vi "PLC.vi"(7 "Notifiers":T4, 8 "error in":errorcluster, 11 "Message Queues":T3) -> (0 "error out":errorcluster)   [LabVIEW 2014]
uses:
  Message Queue/Message Queue.lvlib
  Message Queue/Enqueue Message (Single).vi
  PL Model/PL Model.lvlib
  <vilib>/Utility/error.llb/Error Cluster From Error Code.vi
  Logger/Logger.lvlib
  <vilib>/ErrorRing/Error Ring.xnode
  DAQ/DAQ.lvlib
  TCP/TCP.lvlib
  Exit Notifiers/PLC Notifiers.ctl
  Exit Notifiers/PLC Notifiers.lvlib
  Message Queue/Message Cluster.ctl
  Message Queue/All Message Queues.ctl
  DAQ/TypeDefs/DAQ data.ctl
  controls/PLC Data.ctl
panel:
  in  "PLC Data":T1
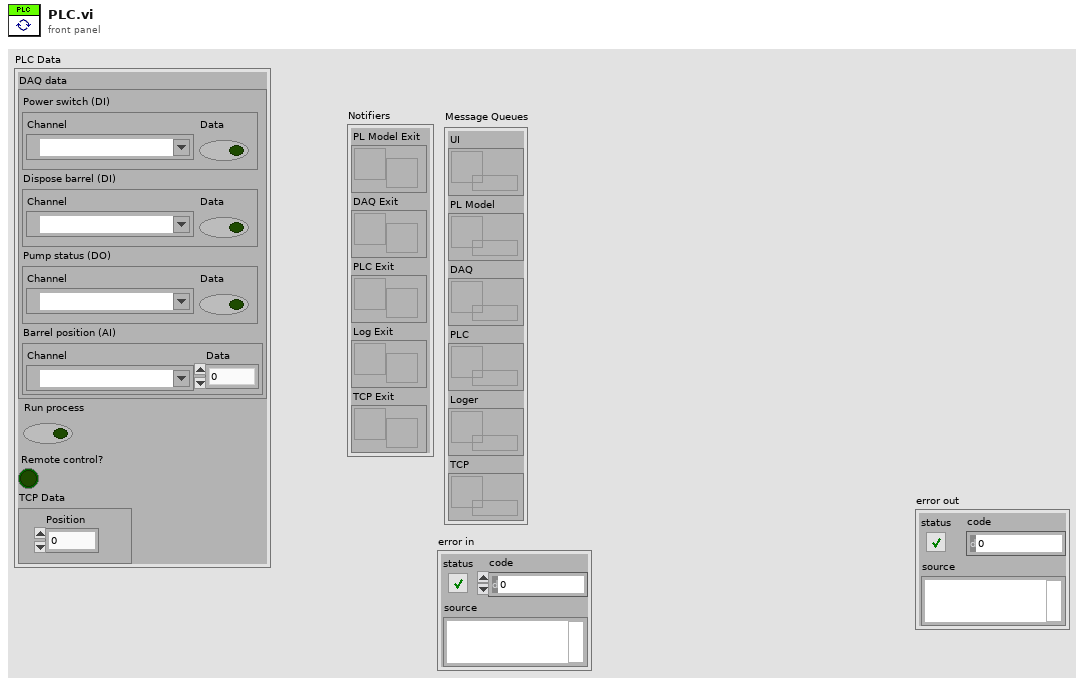
[diagram p1: front panel]
types:
  T1 = typedef "PLC Data.ctl" = cluster{"DAQ data":T2, "Run process":bool, "Remote control?":bool, "TCP Data":cluster{"Position":dbl}}
  T2 = typedef "DAQ.lvlib/DAQ data.ctl" = cluster{"Power switch (DI)":cluster{"Channel":tag, "Data":bool}, "Dispose barrel (DI)":cluster{"Channel":tag, "Data":bool}, "Pump status (DO)":cluster{"Channel":tag, "Data":bool}, "Barrel position (AI)":cluster{"Channel":tag, "Data":dbl}}
  T3 = typedef "Message Queue.lvlib/All Message Queues.ctl" = cluster{"UI":refnum<queue>, "PL Model":refnum<queue>, "DAQ":refnum<queue>, "PLC":refnum<queue>, "Loger":refnum<queue>, "TCP":refnum<queue>}
  T4 = typedef "PLC Notifiers.lvlib/PLC Notifiers.ctl" = cluster{"PL Model Exit":refnum<notifier>, "DAQ Exit":refnum<notifier>, "PLC Exit":refnum<notifier>, "Log Exit":refnum<notifier>, "TCP Exit":refnum<notifier>}
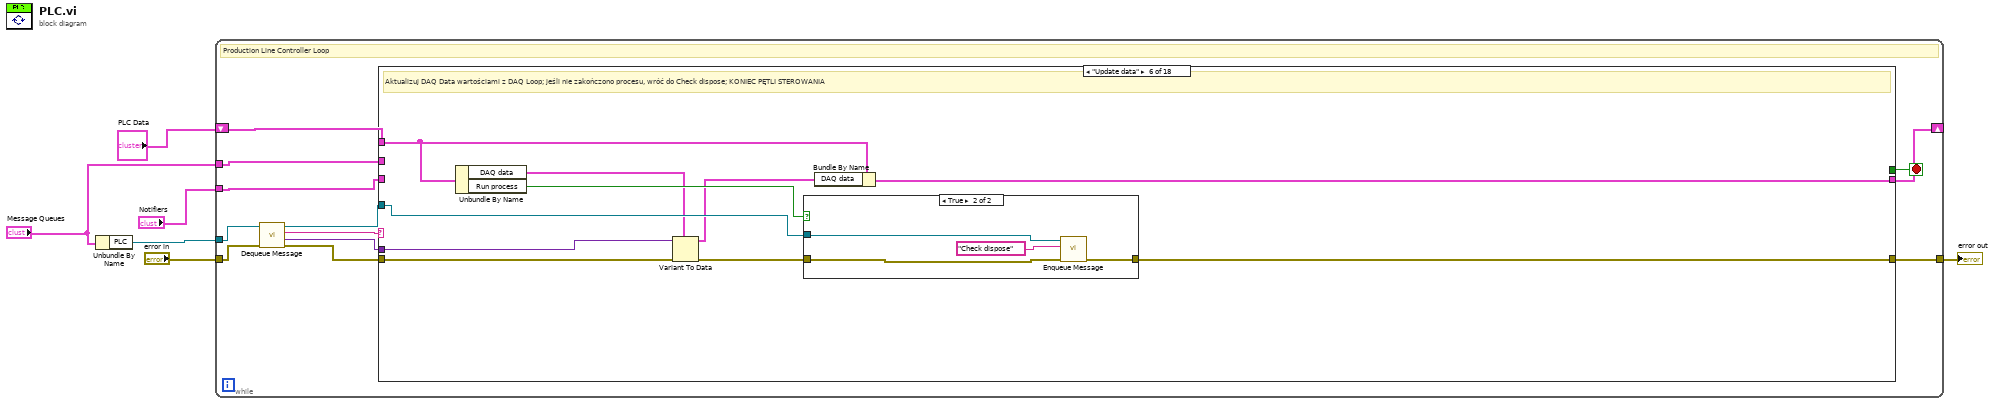
[diagram p0: block diagram]
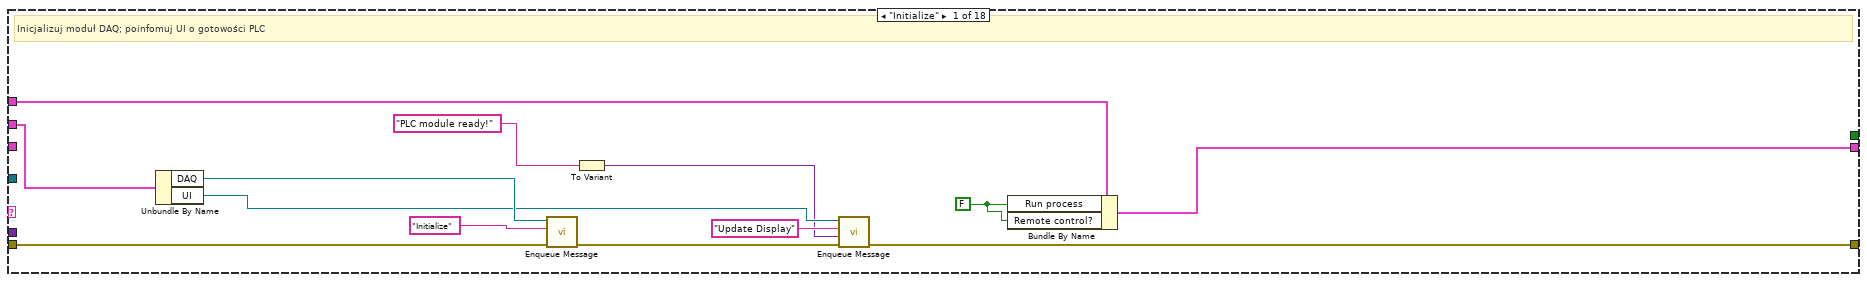
[diagram p2: hidden frame]
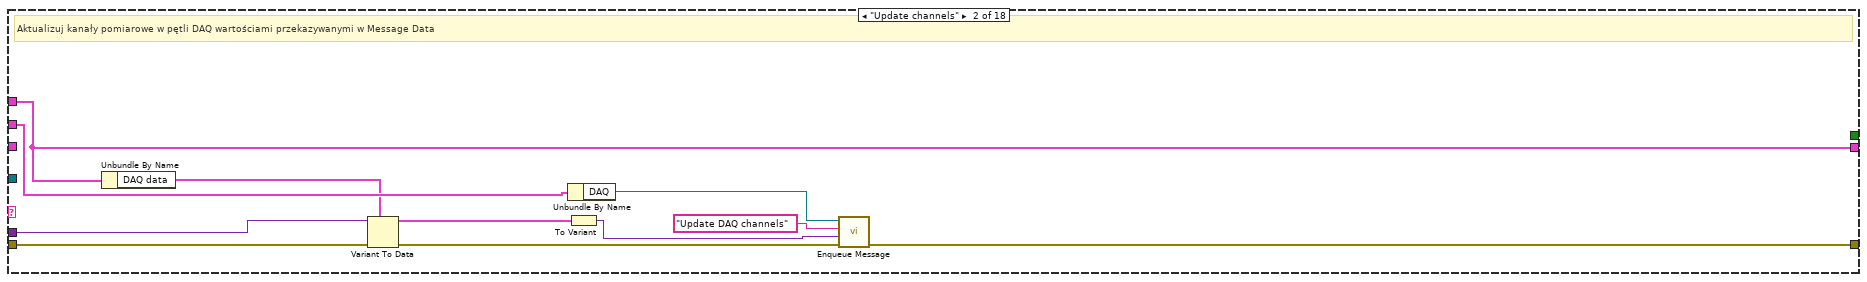
[diagram p3: hidden frame]
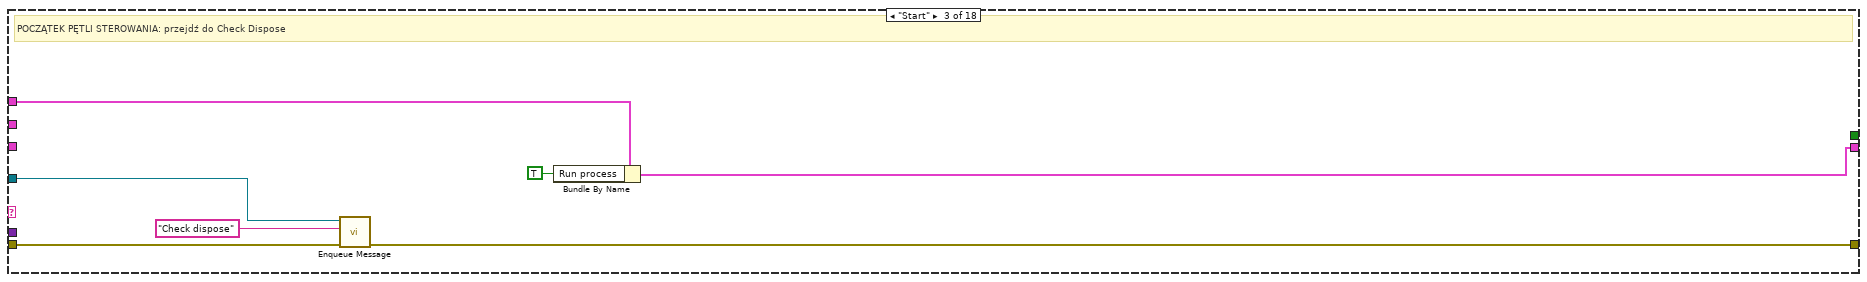
[diagram p4: hidden frame]
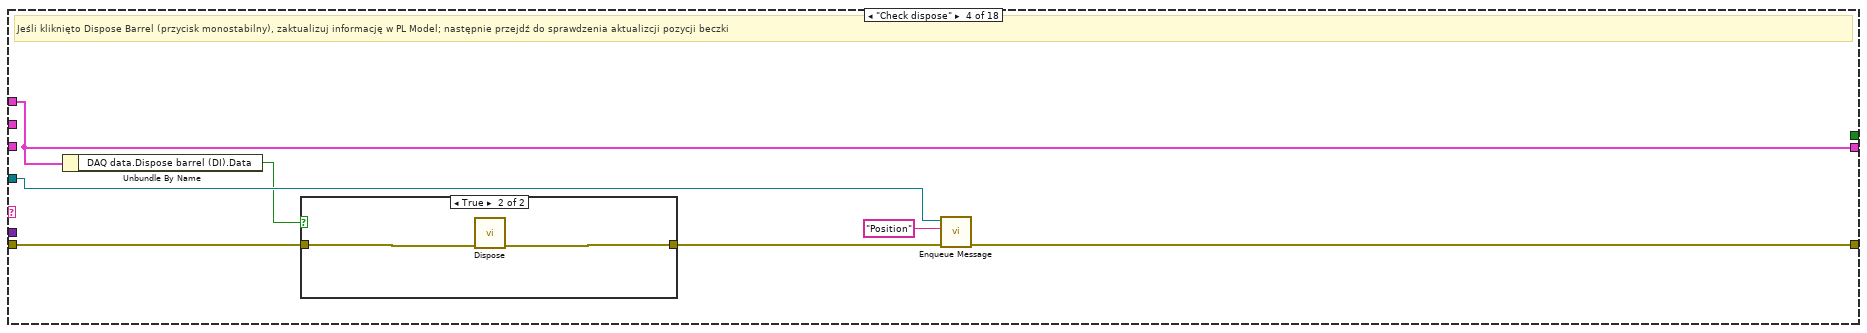
[diagram p5: hidden frame]
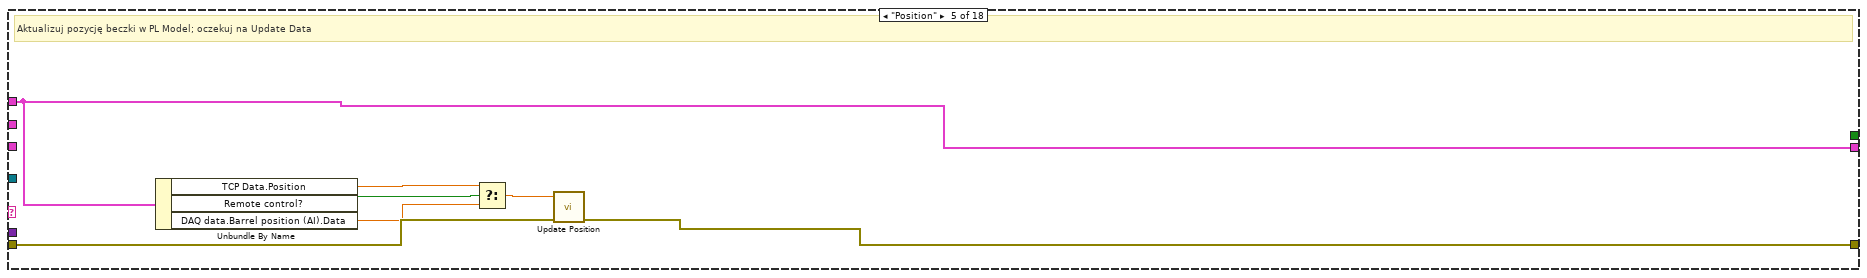
[diagram p7: hidden frame]
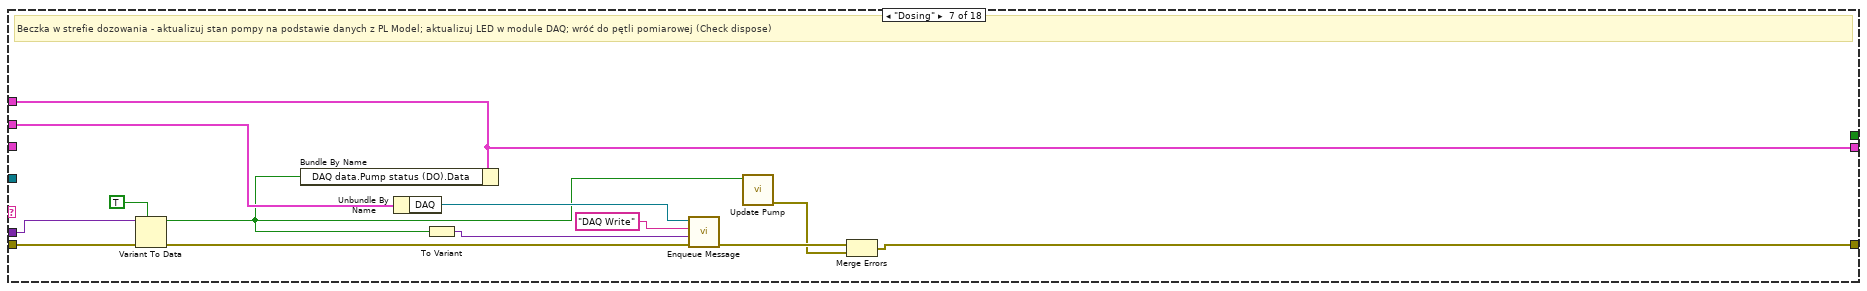
[diagram p9: hidden frame]
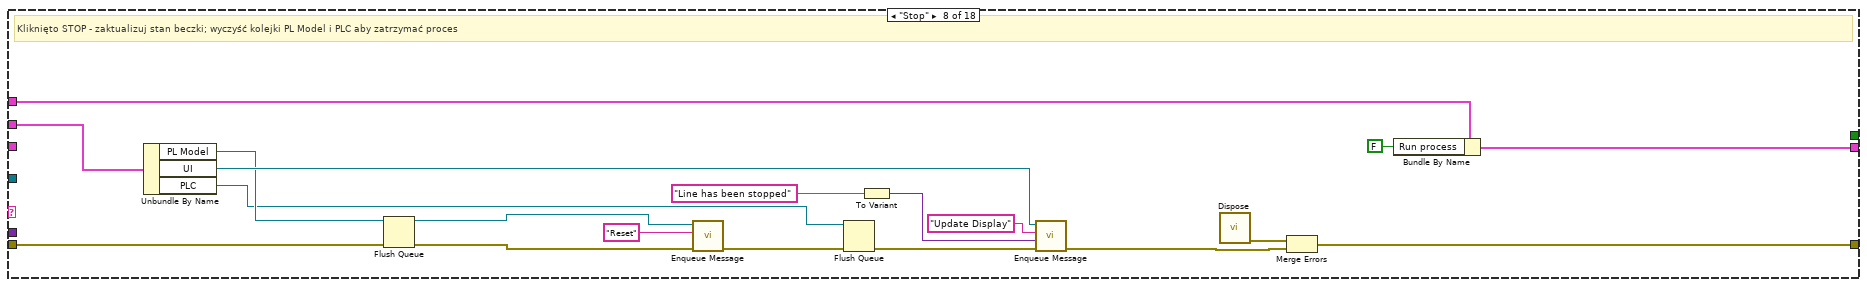
[diagram p10: hidden frame]
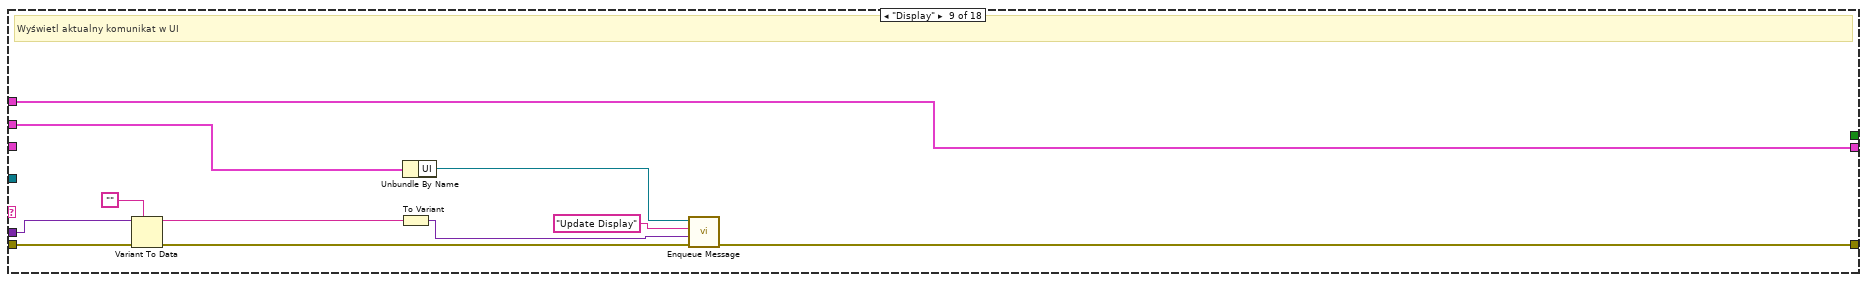
[diagram p11: hidden frame]
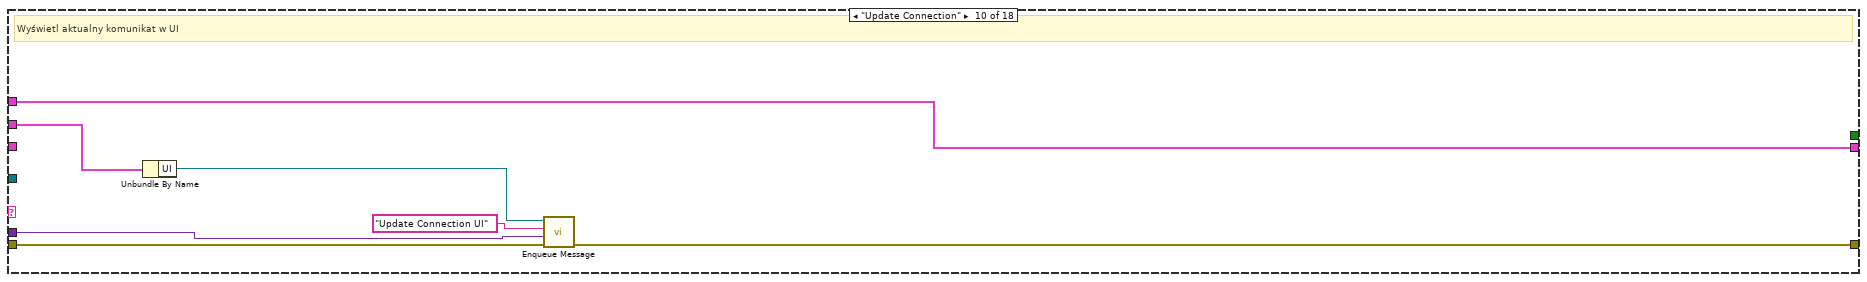
[diagram p12: hidden frame]
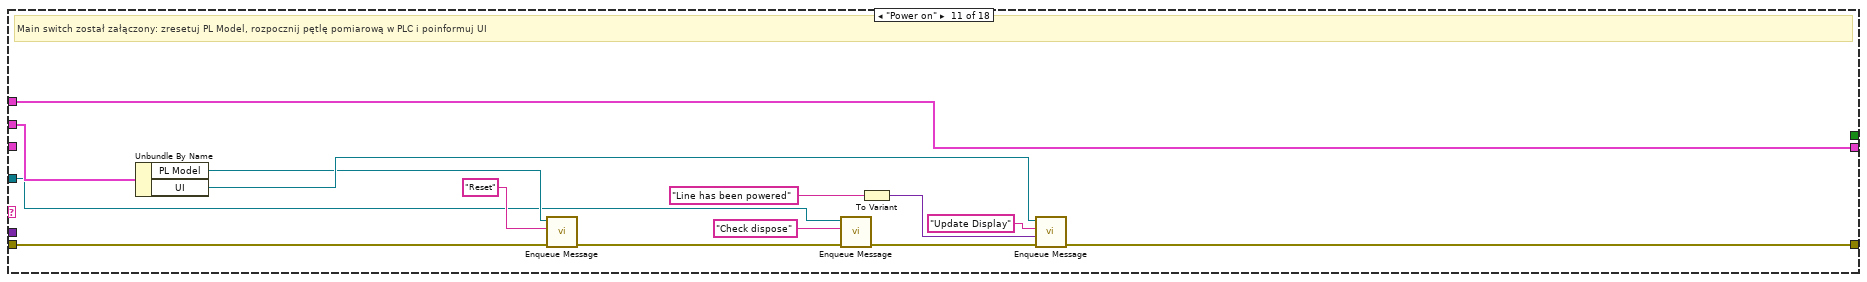
[diagram p13: hidden frame]
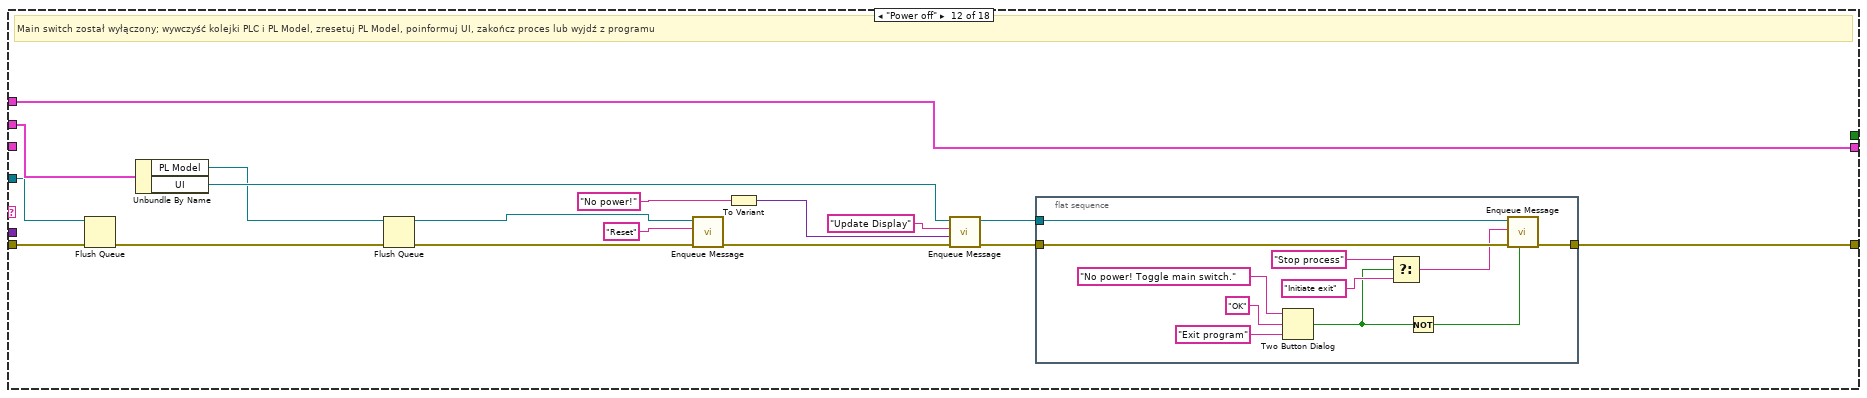
[diagram p14: hidden frame]
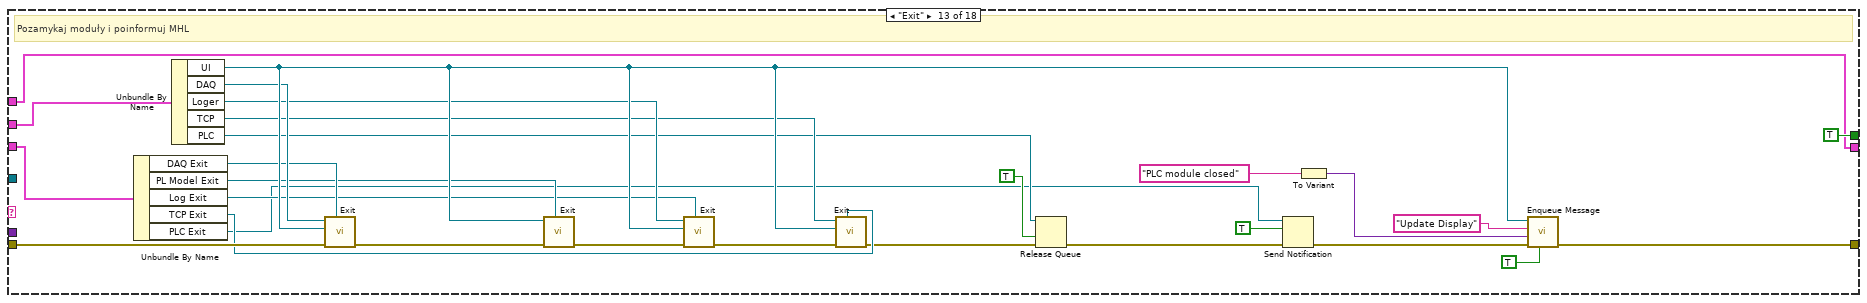
[diagram p15: hidden frame]
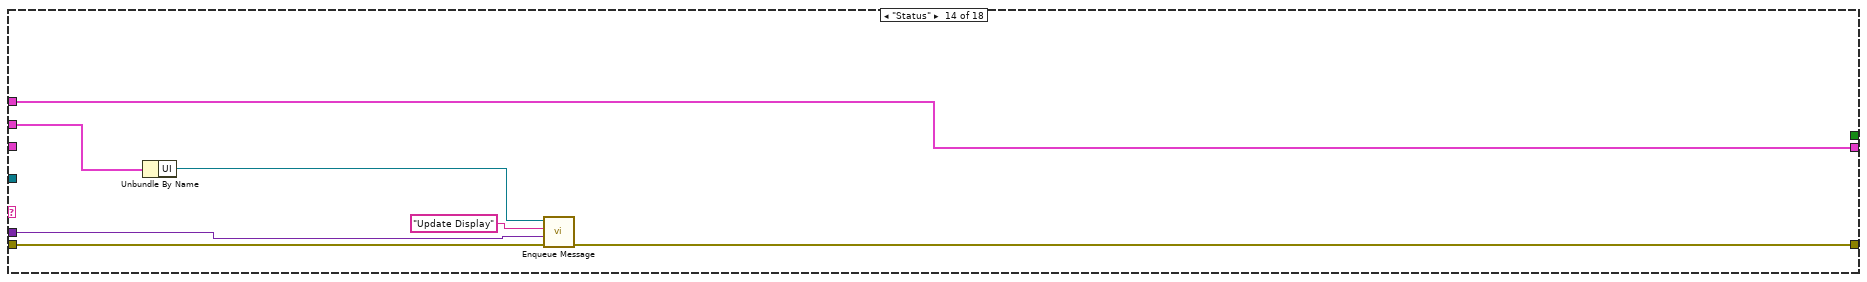
[diagram p16: hidden frame]
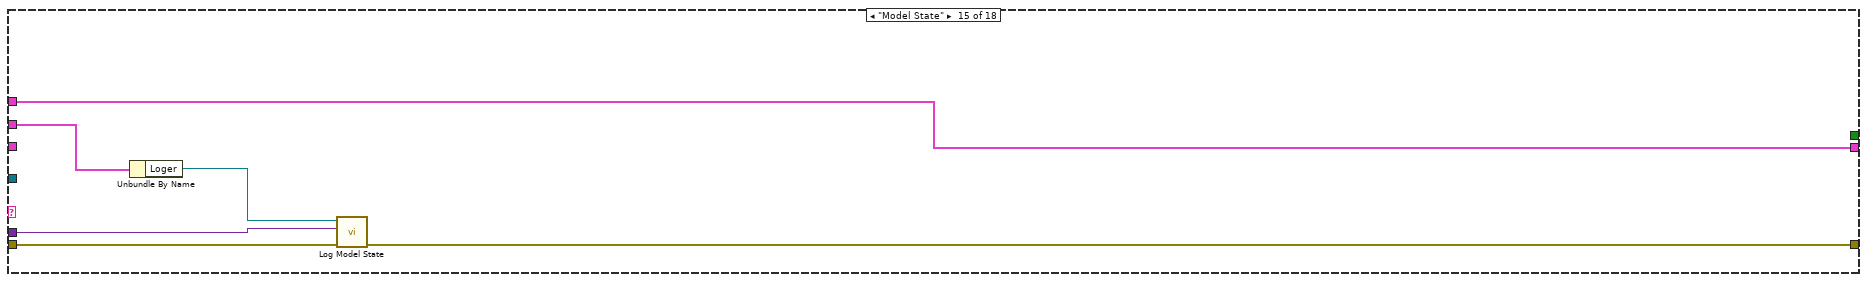
[diagram p17: hidden frame]
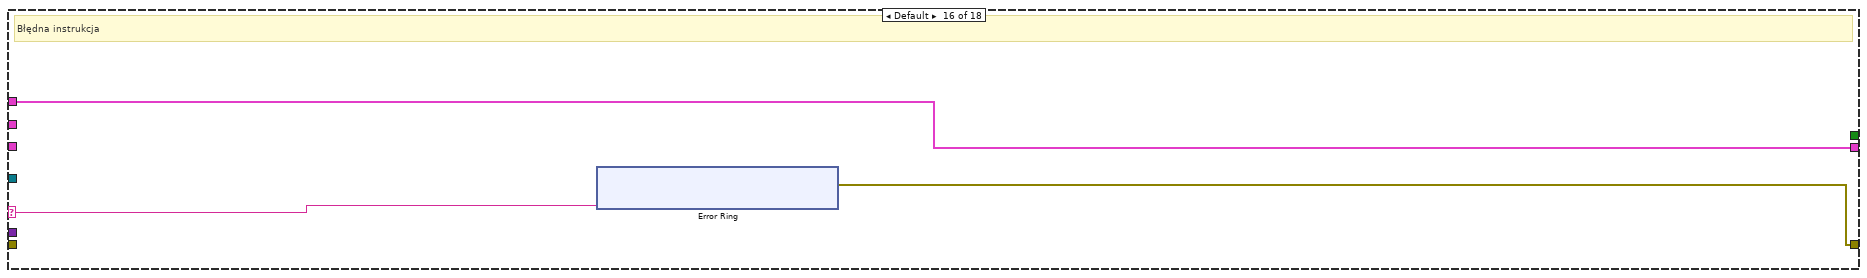
[diagram p18: hidden frame]
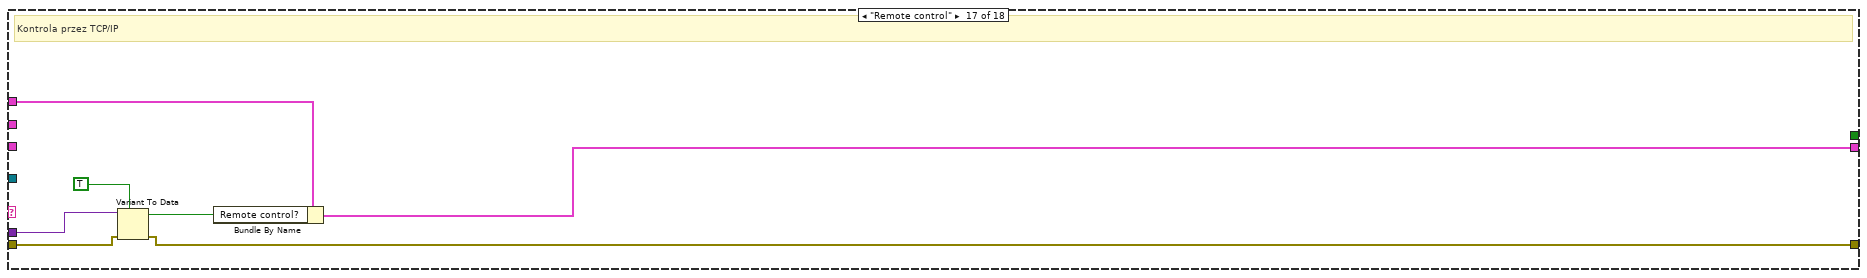
[diagram p19: hidden frame]
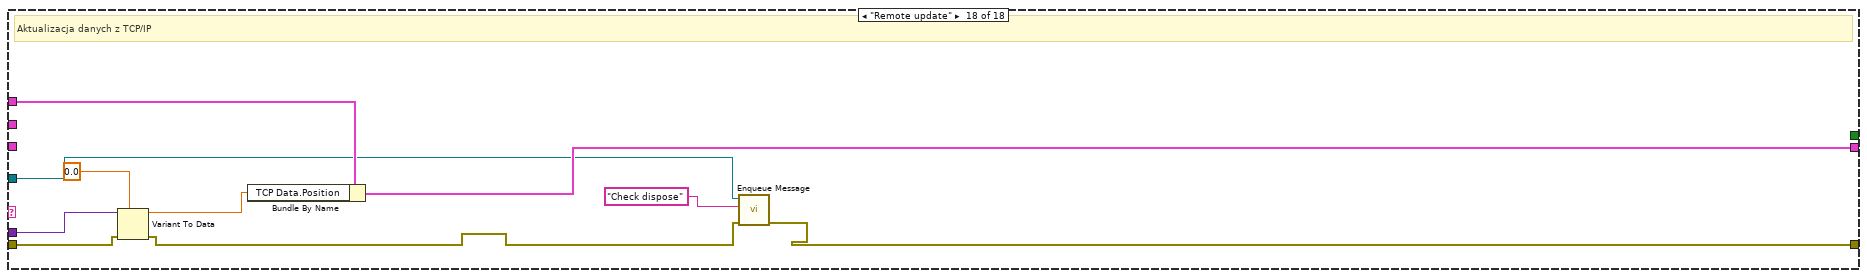
[diagram p20: hidden frame]
diagram:
  n1 = Unbundle By Name("Message Queues") -> ("PLC"=w3:refnum<queue>)
  n2 = while {
    tunnel: "Notifiers" -> [w17]
    tunnel: w3 -> [w16]
    tunnel: "error in" -> [w15]
    tunnel: [w12] -> w5
    tunnel: "Message Queues" -> [w11]
    shift-right: [w9] -> _
    shift-left: "PLC Data" -> [w8]
    stop <- w13 stop-if-true
    # "Production Line Controller Loop"
    n3 = call "Dequeue Message.vi"("error in (no error)"=w15, "Message Queue"=w16) -> ("error out"=w14:errorcluster, "Message Data"=w10:variant, "Message"=w18:string, "dup Message Queue"=w7:refnum<queue>)  [unwired: 6 in]
    n4 = case shown="\"Update data\"" w18 {
      selector: w18 -> [_ _ _ _ _ _ _ _ _ _ _ _ _ _ _ w216 _ _]
      tunnel: w17 -> [_ _ _ _ _ _ _ _ _ _ _ _ w196 _ _ _ _ _]
      tunnel: w14 -> [w30 w41 w43 w53 w66 w75 w90 w109 w120 w125 w139 w153 w199 w206 w211 _ w231 w241]
      tunnel: w7 -> [_ _ w48 w56 _ w74 _ _ _ _ w137 w154 _ _ _ _ _ w232]
      tunnel: [_ _ _ _ _ _ _ _ _ _ _ _ TRUE _ _ _ _ _] -> w13
      tunnel: [w24 w36 w47 w54 w60 w72 w82 w96 w122 w129 w133 w157 w174 w202 w209 w215 w225 w233] -> w12
      tunnel: w11 -> [w31 w38 _ _ _ _ w94 w113 w124 w131 w143 w162 w197 w207 w213 _ _ _]
      tunnel: w10 -> [_ w42 _ _ _ w76 w89 _ w121 w126 _ _ _ w204 w210 _ w230 w240]
      tunnel: w8 -> [w21 w33 w46 w50 w65 w71 w91 w104 w114 w127 w132 w146 w200 w208 w214 w217 w227 w239]
      tunnel: [w20 w33 w45 w50 w65 w70 w91 w102 w114 w127 w132 w146 w200 w208 w214 w217 w226 w238] -> w9
      frame "Initialize" {
        w19 = FALSE ("Run process")
        # "Inicjalizuj moduł DAQ; poinfomuj UI o gotowości PLC"
        n5 = Unbundle By Name(w31) -> ("DAQ"=w29:refnum<queue>, "UI"=w23:refnum<queue>)
        n6 = call-poly "Enqueue Message.vi"("error in (no error)"=w30, "Message"="Initialize", "Message Queue"=w29) -> ("error out"=w25:errorcluster)  [unwired: 7 in, 1 out]
        n7 = To Variant(anything="PLC module ready!" ("Message")) -> (Variant=w22:variant)
        n8 = call-poly "Enqueue Message.vi"("error in (no error)"=w25, "Message Data"=w22, "Message"="Update Display", "Message Queue"=w23) -> ("error out"=w24:errorcluster)  [unwired: 6 in, 1 out]
        n9 = Bundle By Name(cluster=w21, "Run process"=w19, "Remote control?"=w19) -> (w20:T1)
      }
      frame "Update channels" {
        # "Aktualizuj kanały pomiarowe w pętli DAQ wartościami przekazywanymi w Message Data"
        n10 = Unbundle By Name(w33) -> ("DAQ data"=w32:T2)
        n11 = Variant To Data(error in=w41, type=w32, Variant=w42) -> (data=w34:T2, error out=w40:errorcluster)
        n12 = Unbundle By Name(w38) -> ("DAQ"=w37:refnum<queue>)
        n13 = To Variant(anything=w34) -> (Variant=w35:variant)
        n14 = call-poly "Enqueue Message.vi"("error in (no error)"=w40, "Message Data"=w35, "Message"="Update DAQ channels", "Message Queue"=w37) -> ("error out"=w36:errorcluster)  [unwired: 6 in, 1 out]
      }
      frame "Start" {
        # "POCZĄTEK PĘTLI STEROWANIA: przejdź do Check Dispose"
        n15 = call-poly "Enqueue Message.vi"("error in (no error)"=w43, "Message"="Check dispose", "Message Queue"=w48) -> ("error out"=w47:errorcluster)  [unwired: 7 in, 1 out]
        n16 = Bundle By Name(cluster=w46, "Run process"=TRUE) -> (w45:T1)
      }
      frame "Check dispose" {
        # "Jeśli kliknięto Dispose Barrel (przycisk monostabilny), zaktualizuj informację w PL Model; następnie przejdź do sprawdzenia aktualizcji pozycji beczki"
        n17 = Unbundle By Name(w50) -> ("DAQ data.Dispose barrel (DI).Data"=w51:bool)
        n18 = case shown="True" w51 {
          tunnel: w53 -> [w57 w59]
          tunnel: [w57 w58] -> w52
          frame False {
          }
          frame True {
            n19 = call "Dispose.vi"("error in (no error)"=w59) -> ("error out"=w58:errorcluster)  [unwired: 10 in]
          }
        }
        n20 = call-poly "Enqueue Message.vi"("error in (no error)"=w52, "Message"="Position", "Message Queue"=w56) -> ("error out"=w54:errorcluster)  [unwired: 7 in, 1 out]
      }
      frame "Position" {
        # "Aktualizuj pozycję beczki w PL Model; oczekuj na Update Data"
        n21 = Unbundle By Name(w65) -> ("TCP Data.Position"=w64:dbl, "Remote control?"=w61:bool, "DAQ data.Barrel position (AI).Data"=w62:dbl)
        n22 = Select(t=w64, s=w61, f=w62) -> (s? t:f=w63:dbl)
        n23 = call "Update Position.vi"("error in (no error)"=w66, "Position"=w63) -> ("error out"=w60:errorcluster)  [unwired: 9 in]
      }
      frame "Update data" {
        # "Aktualizuj DAQ Data wartościami z DAQ Loop; jeśli nie zakończono procesu, wróć do Check dispose; KONIEC PĘTLI STEROWANIA"
        n24 = Unbundle By Name(w71) -> ("DAQ data"=w67:T2, "Run process"=w69:bool)
        n25 = Variant To Data(error in=w75, type=w67, Variant=w76) -> (data=w68:T2, error out=w73:errorcluster)
        n26 = case shown="True" w69 {
          tunnel: w74 -> [_ w80]
          tunnel: w73 -> [w77 w79]
          tunnel: [w77 w78] -> w72
          frame False {
          }
          frame True {
            n27 = call-poly "Enqueue Message.vi"("error in (no error)"=w79, "Message"="Check dispose", "Message Queue"=w80) -> ("error out"=w78:errorcluster)  [unwired: 7 in, 1 out]
          }
        }
        n28 = Bundle By Name(cluster=w71, "DAQ data"=w68) -> (w70:T1)
      }
      frame "Dosing" {
        # "Beczka w strefie dozowania - aktualizuj stan pompy na podstawie danych z PL Model; aktualizuj LED w module DAQ; wróć do pętli pomiarowej (Check dispose)"
        n29 = Variant To Data(error in=w90, type=TRUE, Variant=w89) -> (data=w86:bool, error out=w83:errorcluster)
        n30 = Bundle By Name(cluster=w91, "DAQ data.Pump status (DO).Data"=w86) -> ()  [unwired: 1 out]
        n31 = Unbundle By Name(w94) -> ("DAQ"=w93:refnum<queue>)
        n32 = To Variant(anything=w86) -> (Variant=w87:variant)
        n33 = call-poly "Enqueue Message.vi"("error in (no error)"=w83, "Message Data"=w87, "Message"="DAQ Write", "Message Queue"=w93) -> ("error out"=w85:errorcluster)  [unwired: 6 in, 1 out]
        n34 = call "Update Pump.vi"("Pump State"=w86) -> ("error out"=w84:errorcluster)  [unwired: 10 in]
        n35 = Merge Errors(w85, w84) -> (w82:errorcluster)
      }
      frame "Stop" {
        # "Kliknięto STOP - zaktualizuj stan beczki; wyczyść kolejki PL Model i PLC aby zatrzymać proces"
        n36 = Unbundle By Name(w113) -> ("PL Model"=w110:refnum<queue>, "UI"=w111:refnum<queue>, "PLC"=w108:refnum<queue>)
        n37 = Flush Queue(queue=w110, error in (no error)=w109) -> (queue out=w101:refnum<queue>, error out=w95:errorcluster)  [unwired: 1 out]
        n38 = call-poly "Enqueue Message.vi"("error in (no error)"=w95, "Message"="Reset", "Message Queue"=w101) -> ("error out"=w99:errorcluster)  [unwired: 7 in, 1 out]
        n39 = Flush Queue(queue=w108, error in (no error)=w99) -> (error out=w107:errorcluster)  [unwired: 2 out]
        n40 = To Variant(anything="Line has been stopped" ("Message")) -> (Variant=w105:variant)
        n41 = call-poly "Enqueue Message.vi"("error in (no error)"=w107, "Message Data"=w105, "Message"="Update Display", "Message Queue"=w111) -> ("error out"=w97:errorcluster)  [unwired: 6 in, 1 out]
        n42 = call "Dispose.vi"() -> ("error out"=w98:errorcluster)  [unwired: 11 in]
        n43 = Merge Errors(w98, w97) -> (w96:errorcluster)
        n44 = Bundle By Name(cluster=w104, "Run process"=FALSE) -> (w102:T1)
      }
      frame "Display" {
        # "Wyświetl aktualny komunikat w UI"
        n45 = Variant To Data(error in=w120, type="", Variant=w121) -> (data=w116:string, error out=w119:errorcluster)
        n46 = To Variant(anything=w116) -> (Variant=w115:variant)
        n47 = Unbundle By Name(w124) -> ("UI"=w123:refnum<queue>)
        n48 = call-poly "Enqueue Message.vi"("error in (no error)"=w119, "Message Data"=w115, "Message"="Update Display", "Message Queue"=w123) -> ("error out"=w122:errorcluster)  [unwired: 6 in, 1 out]
      }
      frame "Update Connection" {
        # "Wyświetl aktualny komunikat w UI"
        n49 = Unbundle By Name(w131) -> ("UI"=w130:refnum<queue>)
        n50 = call-poly "Enqueue Message.vi"("error in (no error)"=w125, "Message Data"=w126, "Message"="Update Connection UI", "Message Queue"=w130) -> ("error out"=w129:errorcluster)  [unwired: 6 in, 1 out]
      }
      frame "Power on" {
        # "Main switch został załączony: zresetuj PL Model, rozpocznij pętlę pomiarową w PLC i poinformuj UI"
        n51 = Unbundle By Name(w143) -> ("PL Model"=w140:refnum<queue>, "UI"=w142:refnum<queue>)
        n52 = call-poly "Enqueue Message.vi"("error in (no error)"=w139, "Message"="Reset", "Message Queue"=w140) -> ("error out"=w136:errorcluster)  [unwired: 7 in, 1 out]
        n53 = call-poly "Enqueue Message.vi"("error in (no error)"=w136, "Message"="Check dispose", "Message Queue"=w137) -> ("error out"=w134:errorcluster)  [unwired: 7 in, 1 out]
        n54 = To Variant(anything="Line has been powered" ("Message")) -> (Variant=w141:variant)
        n55 = call-poly "Enqueue Message.vi"("error in (no error)"=w134, "Message Data"=w141, "Message"="Update Display", "Message Queue"=w142) -> ("error out"=w133:errorcluster)  [unwired: 6 in, 1 out]
      }
      frame "Power off" {
        # "Main switch został wyłączony; wywczyść kolejki PLC i PL Model, zresetuj PL Model, poinformuj UI, zakończ proces lub wyjdź z programu"
        n56 = Flush Queue(queue=w154, error in (no error)=w153) -> (error out=w152:errorcluster)  [unwired: 2 out]
        n57 = Unbundle By Name(w162) -> ("PL Model"=w151:refnum<queue>, "UI"=w161:refnum<queue>)
        n58 = Flush Queue(queue=w151, error in (no error)=w152) -> (queue out=w150:refnum<queue>, error out=w149:errorcluster)  [unwired: 1 out]
        n59 = call-poly "Enqueue Message.vi"("error in (no error)"=w149, "Message"="Reset", "Message Queue"=w150) -> ("error out"=w147:errorcluster)  [unwired: 7 in, 1 out]
        n60 = To Variant(anything="No power!" ("Message")) -> (Variant=w155:variant)
        n61 = call-poly "Enqueue Message.vi"("error in (no error)"=w147, "Message Data"=w155, "Message"="Update Display", "Message Queue"=w161) -> ("error out"=w158:errorcluster, "dup Message Queue"=w156:refnum<queue>)  [unwired: 6 in]
        n62 = flat-sequence {
          tunnel: w158 -> [w170]
          tunnel: [w169] -> w157
          tunnel: w156 -> [w168]
          frame #0 {
            n63 = Two Button Dialog(message="No power! Toggle main switch.", 1:"Exit program" ("F button name (\"Cancel\")"), 2:"OK" ("button name (\"OK\")")) -> (T button?=w164:bool)
            n64 = Select(t="Stop process" ("Message"), s=w164, f="Initiate exit" ("Message")) -> (s? t:f=w165:string)
            n65 = Not(x=w164) -> (.not. x?=w163:bool)
            n66 = call-poly "Enqueue Message.vi"("Priority Message? (F)"=w163, "error in (no error)"=w170, "Message"=w165, "Message Queue"=w168) -> ("error out"=w169:errorcluster)  [unwired: 6 in, 1 out]
          }
        }
      }
      frame "Exit" {
        # "Pozamykaj moduły i poinformuj MHL"
        n67 = Unbundle By Name(w196) -> ("DAQ Exit"=w181:refnum<notifier>, "PL Model Exit"=w180:refnum<notifier>, "Log Exit"=w179:refnum<notifier>, "TCP Exit"=w178:refnum<notifier>, "PLC Exit"=w177:refnum<notifier>)
        n68 = Unbundle By Name(w197) -> ("UI"=w186:refnum<queue>, "DAQ"=w185:refnum<queue>, "Loger"=w184:refnum<queue>, "TCP"=w183:refnum<queue>, "PLC"=w182:refnum<queue>)
        n69 = call "Exit.vi"("Exit Notifier"=w181, "error in"=w199, "UI Queue"=w186, "Message Queue"=w185) -> ("error out"=w195:errorcluster)  [unwired: 7 in]
        n70 = call "Exit.vi"("Exit Notifier"=w180, "error in (no error)"=w195, "UI Queue"=w186) -> ("error out"=w198:errorcluster)  [unwired: 8 in]
        n71 = call "Exit.vi"("Exit Notifier"=w179, "error in (no error)"=w198, "UI Queue"=w186, "Message Queue"=w184) -> ("error out"=w187:errorcluster)  [unwired: 7 in]
        n72 = call "Exit.vi"("Exit Notifier"=w178, "error in"=w187, "UI Queue"=w186, "Message Queue"=w183) -> ("error out"=w176:errorcluster)  [unwired: 7 in]
        n73 = Release Queue(queue=w182, force destroy? (F)=TRUE, error in (no error)=w176) -> (error out=w188:errorcluster)  [unwired: 2 out]
        n74 = Send Notification(notification=TRUE, notifier=w177, error in (no error)=w188) -> (error out=w175:errorcluster)  [unwired: 1 out]
        n75 = To Variant(anything="PLC module closed" ("Message")) -> (Variant=w194:variant)
        n76 = call-poly "Enqueue Message.vi"("Priority Message? (F)"=TRUE, "error in (no error)"=w175, "Message Data"=w194, "Message"="Update Display", "Message Queue"=w186) -> ("error out"=w174:errorcluster)  [unwired: 5 in, 1 out]
      }
      frame "Status" {
        n77 = Unbundle By Name(w207) -> ("UI"=w205:refnum<queue>)
        n78 = call-poly "Enqueue Message.vi"("error in (no error)"=w206, "Message Data"=w204, "Message"="Update Display", "Message Queue"=w205) -> ("error out"=w202:errorcluster)  [unwired: 6 in, 1 out]
      }
      frame "Model State" {
        n79 = Unbundle By Name(w213) -> ("Loger"=w212:refnum<queue>)
        n80 = call "Log Model State.vi"("error in (no error)"=w211, "Message Data"=w210, "Message Queue"=w212) -> ("error out"=w209:errorcluster)  [unwired: 8 in]
      }
      frame Default {
        # "Błędna instrukcja"
        n81 = xnode "Error Ring"("parameter 0"=w216) -> ("error out"=w215:errorcluster)
      }
      frame "Remote control" {
        # "Kontrola przez TCP/IP"
        n82 = Variant To Data(error in=w231, type=TRUE, Variant=w230) -> (data=w228:bool, error out=w225:errorcluster)
        n83 = Bundle By Name(cluster=w227, "Remote control?"=w228) -> (w226:T1)
      }
      frame "Remote update" {
        # "Aktualizacja danych z TCP/IP"
        n84 = Variant To Data(error in=w241, type=0.0, Variant=w240) -> (data=w237:dbl, error out=w234:errorcluster)
        n85 = Bundle By Name(cluster=w239, "TCP Data.Position"=w237) -> (w238:T1)
        n86 = call-poly "Enqueue Message.vi"("error in (no error)"=w234, "Message"="Check dispose", "Message Queue"=w232) -> ("error out"=w233:errorcluster)  [unwired: 7 in, 1 out]
      }
    }
  }
  "error out" <- w5
